vi "Read Climb Operation.vi"(8 "Command Info":T3) -> (0 "Command Info":T3, 1 "SubSystem Data":T1={"Operation"=enum."Read Current", "Setpoint Rhino"=0.0, "Setpoint WHEELS"=0.0, "Roll"=0.0, "Pitch"=0.0, "Reset"=FALSE, "Speedy Tilt"={"Right"=TRUE, "Left"=TRUE}, "Climb"=enum."Level 1-3", "New Pos?"=FALSE, "Defense mode?"=FALSE}, 2 "Command Timing":cluster{"Start Time (ms)":u32, "Iterations":i32})   [LabVIEW 2018]
doc: "This returns the most recently scheduled command. This doesn't indicate whether the command finished and is running the default command."
uses:
  <vilib>/Rock Robotics/WPI/Framework/Command Status Info.ctl
  <vilib>/Rock Robotics/WPI/Framework/Completion Status.ctl
  <vilib>/Rock Robotics/WPI/Framework/Completion Notifier.ctl
  Implementation/Climb Setpoints.ctl
  Implementation/Climb Operations.ctl
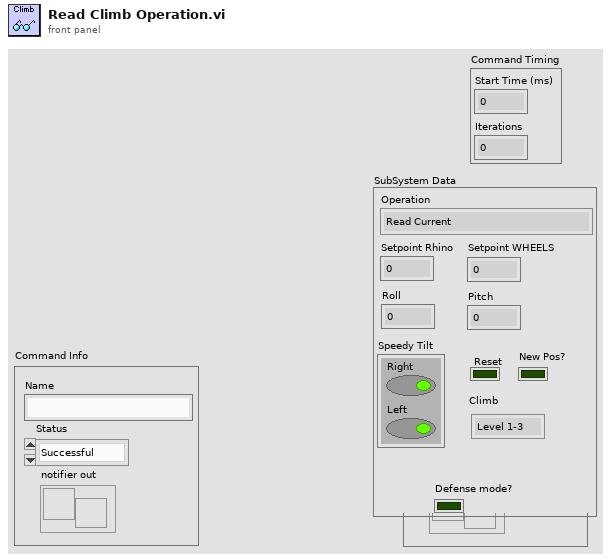
[diagram p1: front panel]
types:
  T1 = typedef "Climb Setpoints.ctl" = cluster{"Operation":T2, "Setpoint Rhino":dbl, "Setpoint WHEELS":dbl, "Roll":dbl, "Pitch":dbl, "Reset":bool, "Speedy Tilt":cluster{"Right":bool, "Left":bool}, "Climb":enum16{"Level 1-3", "Level 1-2", "Level 2-3"}, "New Pos?":bool, "Defense mode?":bool}
  T2 = typedef "Climb Operations.ctl" = enum16{"Reserve", "Read Current", "Immediate", "Ready", "Auto-Climb", "Reset/Turbo-Tilt", "Manual Climb"}
  T3 = typedef "Command Status Info.ctl" = cluster{"Name":string, "Status":T4, "notifier out":T5}
  T4 = typedef "Completion Status.ctl" = enum16{"Successful", "Aborted", "Incomplete"}
  T5 = typedef "Completion Notifier.ctl" = refnum<notifier>
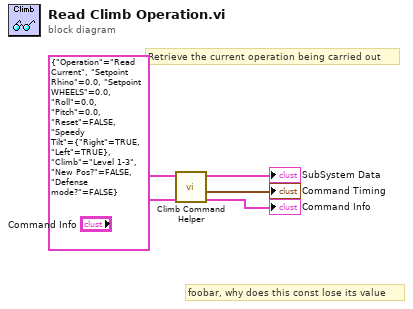
[diagram p0: block diagram]
diagram:
  # "foobar, why does this const lose its value"
  # "Retrieve the current operation being carried out"
  n1 = call "Climb Command Helper.vi"("Command Info In"="Command Info", "SubSystem Data"=T1 {"Operation"=enum."Read Current", "Setpoint Rhino"=0.0, "Setpoint WHEELS"=0.0, "Roll"=0.0, "Pitch"=0.0, "Reset"=FALSE, "Speedy Tilt"={"Right"=TRUE, "Left"=TRUE}, "Climb"=enum."Level 1-3", "New Pos?"=FALSE, "Defense mode?"=FALSE}) -> ("Command Info Out"=→"Command Info":T3, "Command Timing"=→"Command Timing":cluster{"Start Time (ms)":u32, "Iterations":i32}, "SubSystem Data"=→"SubSystem Data":T1)  [unwired: 7 in]
